vi "ReadyToDriveSoundControl.vi"(11 "stop":bool) -> ()   [LabVIEW 2014]
uses:
  <vilib>/FPGAPlugInAG/sbRIO-9626/niLvFpga_Open_sbRIO-9626.vi
  <vilib>/rvi/interface/common/dynamic/niFpgaDynamicAddResources.vi
  Global Data.vi
  <vilib>/Utility/error.llb/Error Cluster From Error Code.vi
  <vilib>/rvi/errors/niLvFpgaAdjustHostInterfaceError.vi
  <vilib>/FPGAPlugInAG/Dynamic/niLvFpga_Close_Dynamic.vi
  <vilib>/rvi/interface/nirviOpenFPGA/nirviOpenFPGA.xnode
  FPGA Bitfiles/FormulaElectric2_FPGATarget_FPGA_KFopRbsiCjk.lvbitx
  FPGA/Sensor Library/FPGA.vi
  <vilib>/rvi/interface/nirviReadWriteControl/nirviReadWriteControl.xnode
  <vilib>/rvi/interface/nirviCloseFPGA/nirviCloseFPGA.xnode
  NiFpgaLv.dll
  <vilib>/rvi/interface/Simulation/niFpgaSimulationCallBeginRW.vi
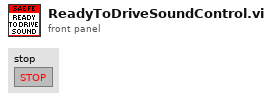
[diagram p1: front panel]
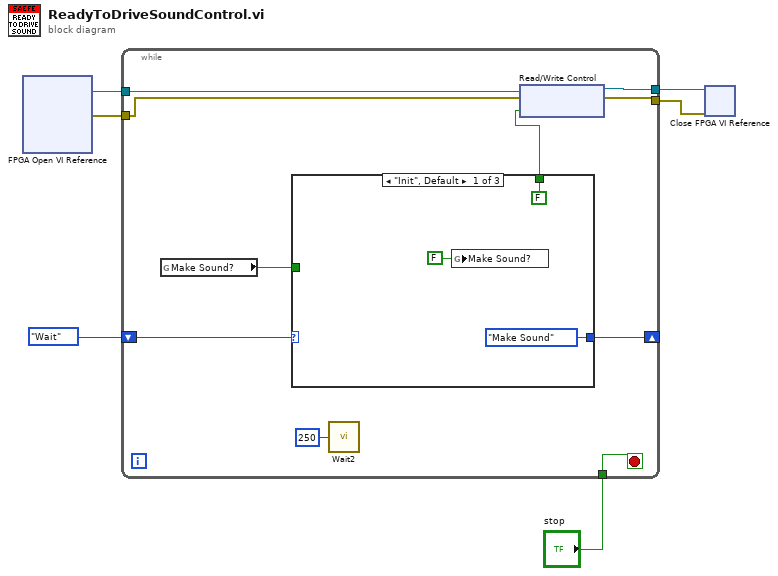
[diagram p0: block diagram]
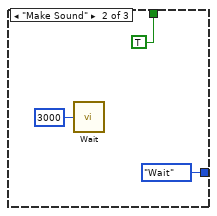
[diagram p2: hidden frame]
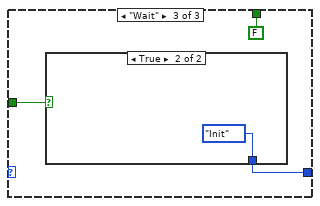
[diagram p3: hidden frame]
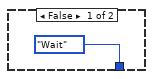
[diagram p4: hidden frame]
diagram:
  n1 = xnode "FPGA Open VI Reference"() -> ("FPGA VI Reference Out"=w4:refnum<k20>, "error out"=w1:errorcluster)  [unwired: 2 in]
  n2 = while {
    tunnel: "stop" -> [w16]
    shift-right: [w9] -> _
    shift-left: enum16{"Init", "Make Sound", "Wait"}."Wait" -> [w11]
    tunnel: w4 -> [w15]
    tunnel: [w14] -> w3
    tunnel: [w13] -> w2
    tunnel: w1 -> [w12]
    stop <- w16 stop-if-true
    n3 = global read "Global Data.vi" "Make Sound?"() -> (w10:bool)
    n4 = case shown="\"Init\", Default" w11 {
      tunnel: w10 -> [_ _ w25]
      tunnel: [enum16{"Init", "Make Sound", "Wait"}."Make Sound" enum16{"Init", "Make Sound", "Wait"}."Wait" w24] -> w9
      tunnel: [FALSE TRUE FALSE] -> w8
      frame "Init", Default {
        n5 = global write "Global Data.vi" "Make Sound?"(FALSE ("Make Sound?")) -> ()
      }
      frame "Make Sound" {
        n6 = call "Wait"("Count(mSec)"=u32 3000) -> ()  [unwired: 1 out]
      }
      frame "Wait" {
        n7 = case shown="True" w25 {
          tunnel: [enum16{"Init", "Make Sound", "Wait"}."Wait" enum16{"Init", "Make Sound", "Wait"}."Init"] -> w24
          frame False {
          }
          frame True {
          }
        }
      }
    }
    n8 = call "Wait2"("Count(mSec)"=u32 250) -> ()  [unwired: 1 out]
    n9 = xnode "Read/Write Control"("FPGA VI Reference In"=w15, "error in"=w12, "RTDS Enable"=w8) -> ("FPGA VI Reference Out"=w14:refnum<k20>, "error out"=w13:errorcluster)
  }
  n10 = xnode "Close FPGA VI Reference"("FPGA VI Reference In"=w3, "error in"=w2) -> ()  [unwired: 1 out]
